vi "WLAN - TxMeasure - Test.vi"() -> ()   [LabVIEW 2012]
uses:
  TV/RW/Includes/WLAN - TV - RW - INC - Tx_IQModResult.ctl
  TV/RW/Includes/WLAN - NIStandardDefine.ctl
panel:
  in  "NIStandard":T1=enum."80211B/G(DSSS)"
  out "Margin VECTOR":dbl[](array[numeric])
  out "Mod Result":T2
  out "error out 3":errorcluster={"status"=TRUE, "code"=-42926, "source"="Property Node (arg 10) in niWLAN - OPPO - 80211abgnIQMeasurementsSettings.vi->WLAN - niVST - RFSA - Measure.vi->WLAN - OPPO - UUT(Tx).vi"}
  out "error out 2":errorcluster
  out "SMM":dbl
  in  "stop":bool
  in  "RFSA":refnum<k15>="RIO0"
  in  "Path Loss dB":dbl
  in  "Center Frequency(Hz)":dbl=5190000000.0
  in  "Power Level(dBm)":dbl
  in  "Channel Bandwidth(Hz)":dbl=80000000.0
  in  "#Avg":i32=1
  out "error out":errorcluster
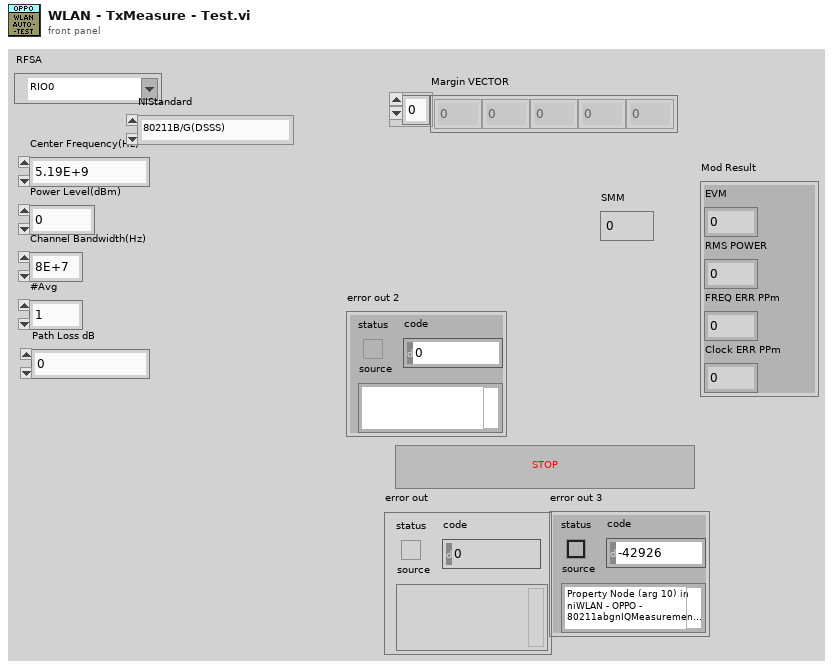
[diagram p1: front panel]
types:
  T1 = typedef "WLAN - NIStandardDefine.ctl" = enum32{"80211A/G/J/P(OFDM)", "80211B/G(DSSS)", "80211GDSSSOFDM", "80211NMIMOOFDM", "80211ACMIMOOFDM"}
  T2 = typedef "WLAN - TV - RW - INC - Tx_IQModResult.ctl" = cluster{"EVM":dbl, "RMS POWER":dbl, "FREQ ERR PPm":dbl, "Clock ERR PPm":dbl}
  T3 = typedef "wlanv1 Analysis Refnum.ctl" = refnum<k20>
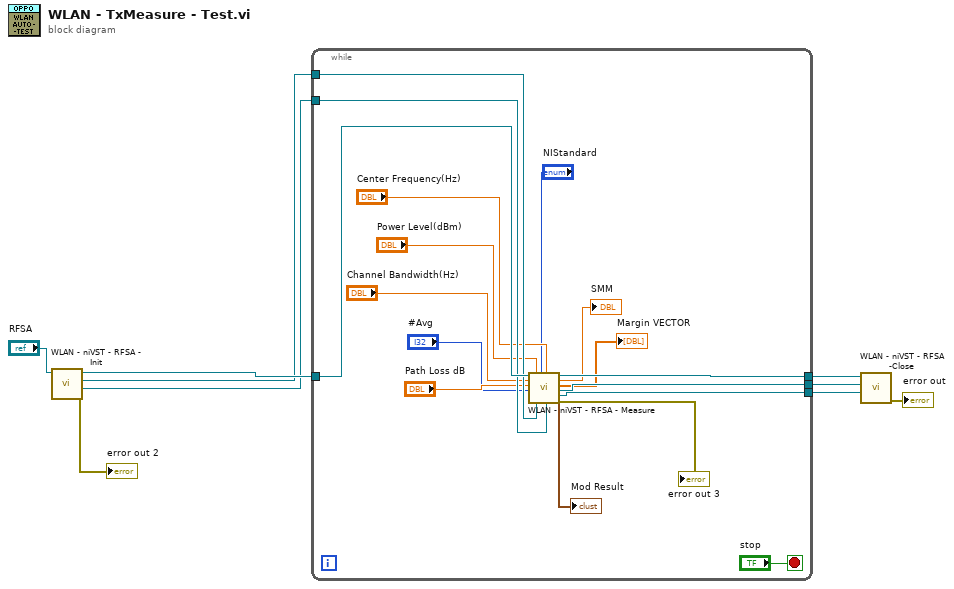
[diagram p0: block diagram]
diagram:
  n1 = call "WLAN - niVST - RFSA - Init.vi"("RFSA Handle"="RFSA") -> ("error out"=→"error out 2":errorcluster, "IQ Measurement Ref"=w5:T3, "Spectrum Meas Ref"=w4:T3, "IVI Refnum out"=w6:refnum<k15>)  [unwired: 7 in]
  n2 = while {
    tunnel: [w26] -> w9
    tunnel: [w25] -> w8
    tunnel: [w24] -> w7
    tunnel: w6 -> [w23]
    tunnel: w5 -> [w22]
    tunnel: w4 -> [w21]
    stop <- "stop" stop-if-true
    n3 = call "WLAN - niVST - RFSA - Measure.vi"("IVI Refnum in"=w23, "Channel Bandwidth(Hz)"="Channel Bandwidth(Hz)", "Path Loss dB"="Path Loss dB", "#Avg"="#Avg", "Power Level(dBm)"="Power Level(dBm)", "Spectrum Meas Ref"=w21, "NIStandard"="NIStandard", "Center Frequency(Hz)"="Center Frequency(Hz)", "IQ Measurement Ref"=w22) -> ("Mod Result"=→"Mod Result":T2, "IVI Refnum out"=w26:refnum<k15>, "SMM"=→"SMM":dbl, "Margin VECTOR"=→"Margin VECTOR":dbl[], "Spectrum Meas Ref out"=w24:T3, "IQ Measurement Ref out"=w25:T3, "error out"=→"error out 3":errorcluster)  [unwired: 4 in]
  }
  n4 = call "WLAN - niVST - RFSA -Close.vi"("IQ Measurement Ref in"=w8, "Spectrum Meas Ref in"=w7, "IVI Refnum in"=w9) -> ("error out"=→"error out":errorcluster)  [unwired: 8 in]
